vi "loadTensorFlowModel.vi"(8 "error in":errorcluster, 11 "Input cluster":T1) -> (0 "error out":errorcluster, 3 "Output cluster":T1)   [LabVIEW 2020]
uses:
  controls/StateMachineVariables.ctl
  <vilib>/vision/Avi.llb/IMAQ AVI2 Refnum.ctl
  <vilib>/userDefined/High Color/IMAQdx.ctl
  <vilib>/vision/Deep Learning.llb/IMAQ DL Model Refnum.ctl
  <vilib>/vision/Image Controls.llb/IMAQ Image.ctl
  <vilib>/vision/Deep Learning.llb/IMAQ DL Model Type.ctl
  <vilib>/vision/NI_Vision_Development_Module.lvlib
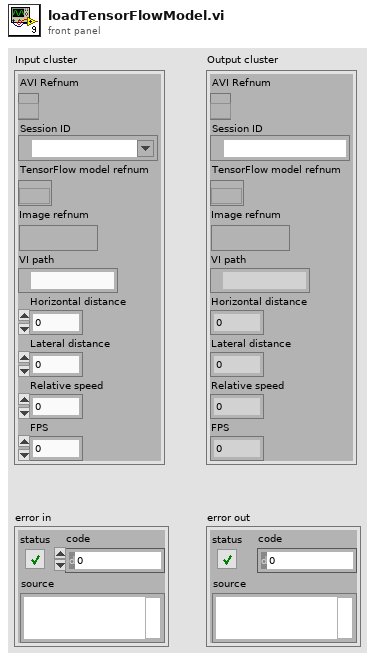
[diagram p1: front panel]
types:
  T1 = typedef "StateMachineVariables.ctl" = cluster{"AVI Refnum":T2, "Session ID":T3, "TensorFlow model refnum":T4, "Image refnum":T5, "VI path":path, "Horizontal distance":dbl, "Lateral distance":dbl, "Relative speed":dbl, "FPS":dbl}
  T2 = typedef "IMAQ AVI2 Refnum.ctl" = refnum<k20>
  T3 = typedef "IMAQdx.ctl" = refnum<k21>
  T4 = typedef "IMAQ DL Model Refnum.ctl" = refnum<k20>
  T5 = typedef "IMAQ Image.ctl" = refnum<image>
  T6 = typedef "IMAQ DL Model Type.ctl" = i32
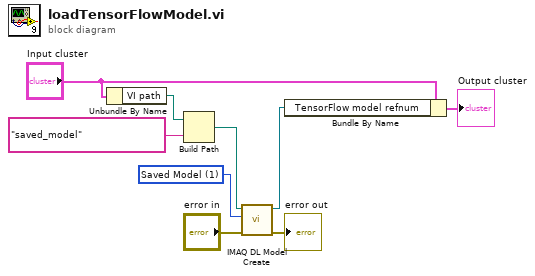
[diagram p0: block diagram]
diagram:
  w9 = T6 1 items=["Frozen Graph", "Saved Model"] ("Model Type")
  n1 = Unbundle By Name("Input cluster") -> ("VI path"=w3:path)
  n2 = Build Path(base path=w3, name or relative path="saved_model") -> (appended path=w7:path)
  n3 = call-poly "IMAQ DL Model Create"("error in (no error)"="error in", "Model Type"=w9, "File Path"=w7) -> ("error out"=→"error out":errorcluster, "Model Refnum"=w4:T4)  [unwired: 7 in]
  n4 = Bundle By Name(cluster="Input cluster", "TensorFlow model refnum"=w4) -> (→"Output cluster":T1)
